vi "BRig_dataLick_iState__afterLick.vi"() -> (2 "output_iState__afterLick":i32)   [LabVIEW 2014]
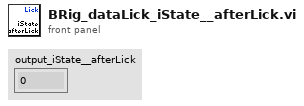
[diagram p1: front panel]
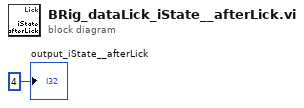
[diagram p0: block diagram]
diagram:
  "output_iState__afterLick" <- 4 ("output_iBlock")
